vi "Autonomous Independent.vi"() -> ()   [LabVIEW 2014]
doc: "This VI is called when autonomous begins, and will automatically be terminated when autonomous ends. You can carry out timed or sensor driven robot movement independently without needing to return to the caller."
uses:
  Command Type.ctl
  <vilib>/Rock Robotics/WPI/RobotDrive/WPI_RobotDriveDevRef.ctl
  <vilib>/Rock Robotics/WPI/MotorControl/WPI_MotorControlDeviceRef.ctl
  <vilib>/Rock Robotics/WPI/MotorControl/WPI_MotorControlType.ctl
  <vilib>/Rock Robotics/SystemInterfaces/Typedef/FPGA_TypedefDigitalModule.ctl
  <vilib>/Rock Robotics/SystemInterfaces/DIO/FPGA_DIOPWMChannel.ctl
  <vilib>/Rock Robotics/WPI/PWM/WPI_PWMDeadband.ctl
  <vilib>/Rock Robotics/WPI/CAN/Jaguar/SubVIs/WPI_CANJaguar_ControlMode.ctl
  <vilib>/Rock Robotics/WPI/CAN/TalonSRX/WPI_CANTalonSRX_APIControlMode.ctl
  <vilib>/Rock Robotics/WPI/PWM/WPI_PWMTransform_ConPane.ctl
  <vilib>/Rock Robotics/WPI/Encoder/WPI_EncoderDevRef.ctl
  <vilib>/Rock Robotics/SystemInterfaces/Encoder/FPGA_EncoderIdx.ctl
  <vilib>/Rock Robotics/SystemInterfaces/Counter/FPGA_CounterCtrSystemIndex.ctl
  <vilib>/Rock Robotics/WPI/Encoder/WPI_EncoderType.ctl
  Nav6Library/Nav6DevRef.ctl
  <vilib>/Rock Robotics/WPI/SerialPort/WPI_SerialPortRef.ctl
  Nav6Library/Nav6Mode.ctl
  <vilib>/addons/control/pid/pid.llb/PID Structure.ctl
  <vilib>/Rock Robotics/WPI/RobotDrive/WPI_RobotDriveGetSetRefNum.vi
  <vilib>/Rock Robotics/Network Tables/SD Read Number.vi
  Robot Global Data.vi
  <vilib>/Rock Robotics/Network Tables/SD Write String.vi
  <vilib>/addons/control/pid/pid.llb/PID (DBL).vi
  GyroGlobal.vi
  <vilib>/addons/control/pid/NI_PID_pid.lvlib
  Nav6Library/Nav6.lvlib
  <vilib>/addons/control/pid/pid.llb/PID Structure Conversion (DBL).vi
  <vilib>/ptbypt/NI_PtbyPt.lvlib
panel:
  in  "stop 3":bool
  out "Outputs 2":dbl(graph)
  in  "Auton Routines":T1[](array[typedef])
  in  "Debug":bool
  in  "stop 2":bool
  in  "stop":bool
  out "Encoders":cluster{dbl, "Distance":dbl, "Distance":dbl}(graph)
  out "Outputs":T2(graph)
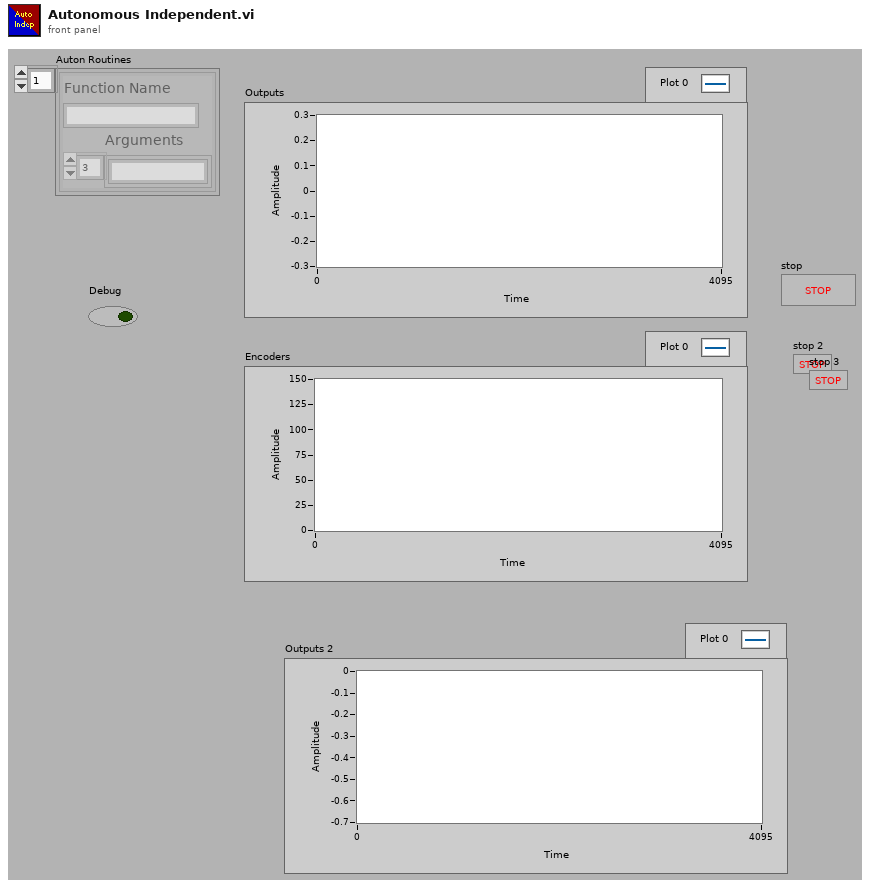
[diagram p1: front panel]
types:
  T1 = typedef "Command Type.ctl" = cluster{"Function Name":string, "Arguments":string[]}
  T2 = cluster{"Motor Values[0]":dbl, "Motor Values[1]":dbl}
  T3 = typedef "WPI_RobotDriveDevRef.ctl" = cluster{"DevStatus":errorcluster, "Motors[]":T4[], "Square Inputs":bool, "Max Output":dbl}
  T4 = typedef "WPI_MotorControlDeviceRef.ctl" = cluster{"DeviceStatus":errorcluster, "Type":T5, "PWM":cluster{"Controller":T6, "PWM Channel":T7, "DeadBand":T8}, "CAN":cluster{"Device Number":u8, "Control Mode":T9, "Semaphore":T10, "Max Vout":dbl, "TalonSRX Control Mode":T11}, "Invert":bool, "TransformRef":T12, "InvTransformRef":T12}
  T5 = typedef "WPI_MotorControlType.ctl" = enum16{"PWM", "CAN", "CANTalonSRX"}
  T6 = typedef "FPGA_TypedefDigitalModule.ctl" = enum16{"Controller 1"}
  T7 = typedef "FPGA_DIOPWMChannel.ctl" = enum8{"PWM 0", "PWM 1", "PWM 2", "PWM 3", "PWM 4", "PWM 5", "PWM 6", "PWM 7", "PWM 8", "PWM 9", "PWM MXP 0", "PWM MXP 1", "PWM MXP 2", "PWM MXP 3", "PWM MXP 4", "PWM MXP 5", "PWM MXP 6", "PWM MXP 7", "PWM MXP 8", "PWM MXP 9", "Invalid"}
  T8 = typedef "WPI_PWMDeadband.ctl" = cluster{"Name":string, "maxPositivePwm":i32, "minPositivePwm":i32, "centerPwm":i32, "maxNegativePwm":i32, "minNegativePwm":i32, "angularRange":u16}
  T9 = typedef "WPI_CANJaguar_ControlMode.ctl" = enum8{"Percent VBus", "Current", "Speed", "Position", "Voltage"}
  T10 = typedef "Semaphore RefNum" = refnum<k1>
  T11 = typedef "WPI_CANTalonSRX_APIControlMode.ctl" = enum8{"Percent VBus", "Speed", "Position", "Slave", "Unchanged / Invalid"}
  T12 = typedef "WPI_PWMTransform_ConPane.ctl" = refnum<vi>
  T13 = typedef "WPI_EncoderDevRef.ctl" = cluster{"DevStatus":errorcluster, "EncoderIndex":T14, "CounterIndex":T15, "DistancePerCount":dbl, "Decoding Type":T16}
  T14 = typedef "FPGA_EncoderIdx.ctl" = enum8{"Enc 0", "Enc 1", "Enc 2", "Enc 3", "Enc 4", "Enc 5", "Enc 6", "Enc 7", "Invalid"}
  T15 = typedef "FPGA_CounterCtrSystemIndex.ctl" = enum8{"Ctr 0", "Ctr 1", "Ctr 2", "Ctr 3", "Ctr 4", "Ctr 5", "Ctr 6", "Ctr 7", "Invalid"}
  T16 = typedef "WPI_EncoderType.ctl" = enum16{"1x", "2x", "4x"}
  T17 = typedef "Nav6.lvlib/Nav6DevRef.ctl" = cluster{"SerialPortRef":T18, "UpdateRate":u8, "Error":errorcluster, "Nav6Mode":T19}
  T18 = typedef "WPI_SerialPortRef.ctl" = cluster{"DevStatus":errorcluster, "Serial Port Name":refnum<visa-resource-name>}
  T19 = typedef "Nav6.lvlib/Nav6Mode.ctl" = enum16{"YPR", "Gyro", "Quaternion"}
  T20 = cluster{"Motors":T3, "EncoderR":T13, "EncoderL":T13, "Nav6":T17}
  T21 = typedef "NI_PID_pid.lvlib/PID Structure.ctl" = u16
  T22 = cluster{"proportional gain (Kc)":dbl, "integral time (Ti, min)":dbl, "derivative time (Td, min)":dbl}
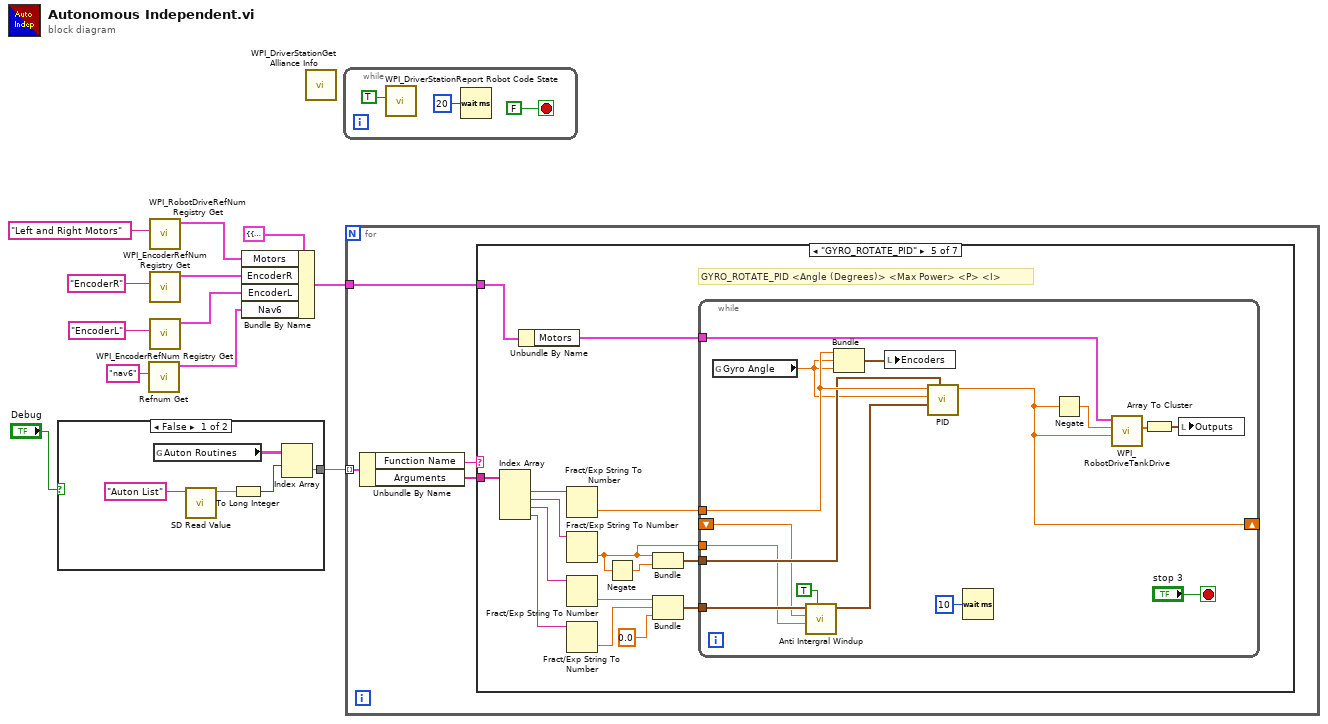
[diagram p0: block diagram]
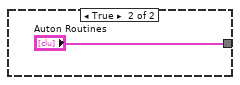
[diagram p2: hidden frame]
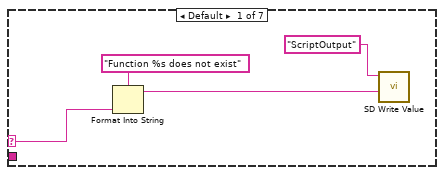
[diagram p3: hidden frame]
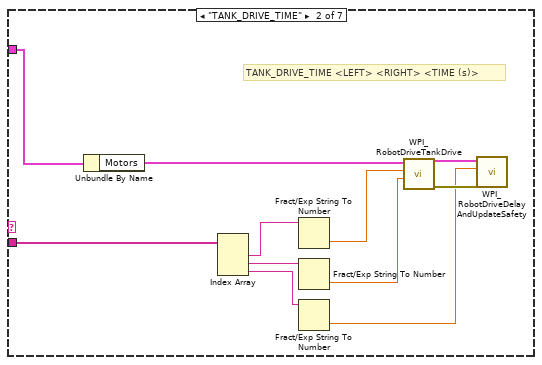
[diagram p4: hidden frame]
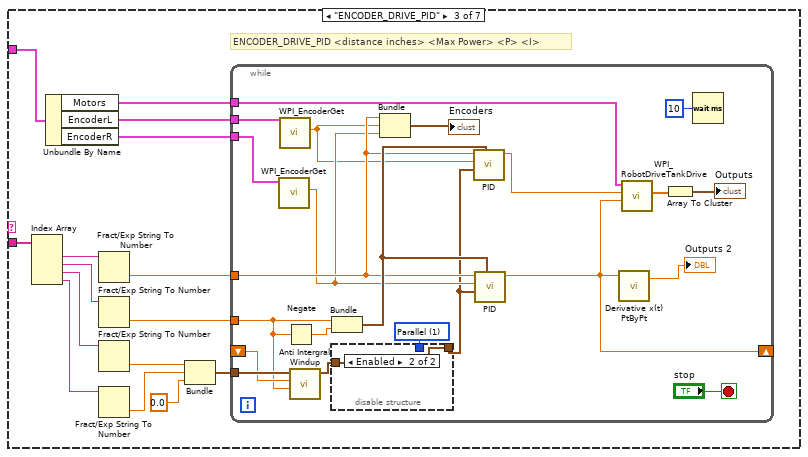
[diagram p5: hidden frame]
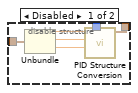
[diagram p6: hidden frame]
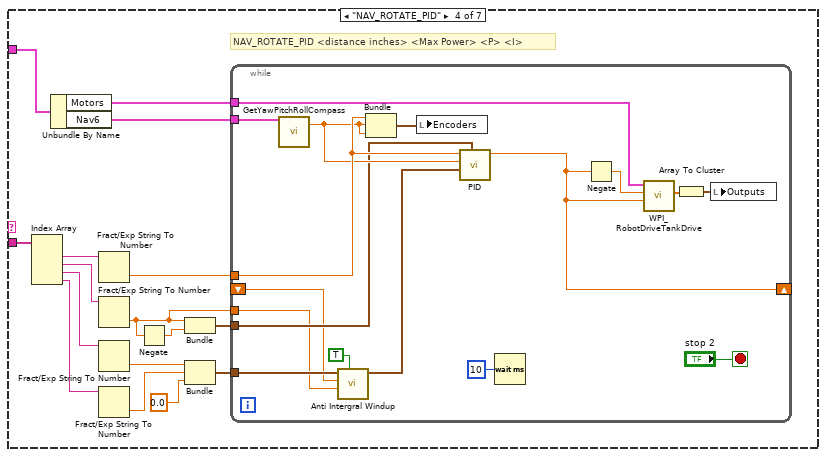
[diagram p7: hidden frame]
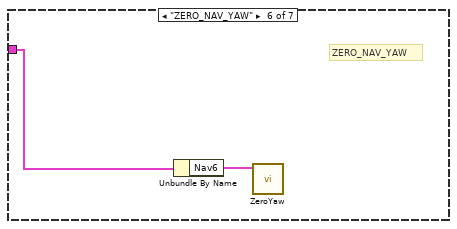
[diagram p8: hidden frame]
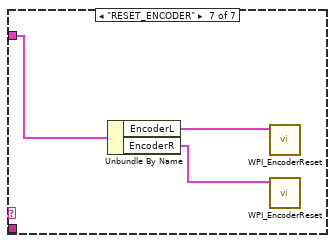
[diagram p9: hidden frame]
diagram:
  n1 = case shown="False" "Debug" {
    tunnel: [w13 "Auton Routines"] -> w12
    frame False {
      n2 = global read "Robot Global Data.vi" "Auton Routines"() -> (w16:T1[][])
      n3 = call-poly <vilib>:"SD Read Value.vi"("Name"="Auton List") -> ("Numeric"=w14:dbl)  [unwired: 8 in, 2 out]
      n4 = To Long Integer(number=w14) -> (32bit integer=w17:i32)
      n5 = Index Array(array=w16, index (row)=w17) -> (element=w13:T1[])  [unwired: 1 in]
    }
    frame True {
    }
  }
  n6 = call "Refnum Get.vi"("refnum name"="nav6") -> ("Nav6DevRef"=w2:T17)  [unwired: 9 in, 1 out]
  n7 = call <vilib>:"WPI_RobotDriveRefNum Registry Get.vi"("refnum name"="Left and Right Motors") -> ("RobotDriveDevRef"=w6:T3)  [unwired: 9 in, 1 out]
  n8 = call <vilib>:"WPI_EncoderRefNum Registry Get.vi"("refnum name"="EncoderR") -> ("EncoderDevRef"=w7:T13)  [unwired: 9 in, 1 out]
  n9 = call <vilib>:"WPI_EncoderRefNum Registry Get.vi"("refnum name"="EncoderL") -> ("EncoderDevRef"=w8:T13)  [unwired: 9 in, 1 out]
  n10 = Bundle By Name(cluster=T20 {"Motors"={"DevStatus"={"status"=FALSE, "code"=0, "source"=""}, "Motors[]"=[], "Square Inputs"=FALSE, "Max Output"=1.0}, "EncoderR"={"DevStatus"={"status"=FALSE, "code"=0, "source"=""}, "EncoderIndex"=enum."Invalid", "CounterIndex"=enum."Invalid", "DistancePerCount"=1.0, "Decoding Type"=enum."4x"}, "EncoderL"={"DevStatus"={"status"=FALSE, "code"=0, "source"=""}, "EncoderIndex"=enum."Invalid", "CounterIndex"=enum."Invalid", "DistancePerCount"=1.0, "Decoding Type"=enum."4x"}, "Nav6"={"SerialPortRef"={"DevStatus"={"status"=FALSE, "code"=0, "source"=""}, "Serial Port Name"=""}, "UpdateRate"=0, "Error"={"status"=FALSE, "code"=0, "source"=""}, "Nav6Mode"=enum."YPR"}}, "Motors"=w6, "EncoderR"=w7, "EncoderL"=w8, "Nav6"=w2) -> (w4:T20)
  n11 = call <vilib>:"WPI_DriverStationGet Alliance Info.vi"() -> ()  [unwired: 12 out]
  n12 = while {
    stop <- FALSE stop-if-true
    n13 = call <vilib>:"WPI_DriverStationReport Robot Code State.vi"("Autonomous"=TRUE) -> ()  [unwired: 10 in, 1 out]
    n14 = Wait (ms)(milliseconds to wait=u32 20) -> ()  [unwired: 1 out]
  }
  n15 = for {
    tunnel: w12 -> [w25] mode=indexing
    tunnel: w4 -> [w22]
    n16 = Unbundle By Name(w25) -> ("Function Name"=w24:string, "Arguments"=w23:string[])
    n17 = case shown="\"GYRO_ROTATE_PID\"" w24 {
      selector: w24 -> [w28 _ _ _ _ _ _]
      tunnel: w23 -> [_ w38 w55 w100 w132 _ _]
      tunnel: w22 -> [_ w31 w50 w96 w128 w150 w153]
      frame Default {
        n18 = Format Into String(format string="Function %s does not exist", w28) -> (resulting string=w26:string)  [unwired: 2 in, 1 out]
        n19 = call-poly <vilib>:"SD Write Value.vi"("String"=w26, "Name"="ScriptOutput") -> ()  [unwired: 8 in, 2 out]
      }
      frame "TANK_DRIVE_TIME" {
        # "TANK_DRIVE_TIME <LEFT> <RIGHT> <TIME (s)>"
        n20 = Unbundle By Name(w31) -> ("Motors"=w30:T3)
        n21 = Index Array(array=w38) -> (element #1=w37:string, element #2=w36:string, element #3=w35:string)  [unwired: 3 in]
        n22 = Fract/Exp String To Number(string=w37) -> (number=w34:dbl)  [unwired: 3 in, 1 out]
        n23 = Fract/Exp String To Number(string=w36) -> (number=w33:dbl)  [unwired: 3 in, 1 out]
        n24 = Fract/Exp String To Number(string=w35) -> (number=w32:dbl)  [unwired: 3 in, 1 out]
        n25 = call <vilib>:"WPI_RobotDriveTankDrive.vi"("Right axis value"=w33, "Left axis value"=w34, "RobotDriveDevRef"=w30) -> ("error out"=w40:errorcluster, "RobotDriveDevRef"=w39:T3)  [unwired: 6 in, 1 out]
        n26 = call <vilib>:"WPI_RobotDriveDelayAndUpdateSafety.vi"("error in (no error)"=w40, "Delay (s)"=w32, "RobotDriveDevRef"=w39) -> ()  [unwired: 7 in, 2 out]
      }
      frame "ENCODER_DRIVE_PID" {
        # "ENCODER_DRIVE_PID <distance inches> <Max Power> <P> <I>"
        n27 = Index Array(array=w55) -> (element #1=w53:string, element #2=w54:string, element #3=w46:string, element #4=w45:string)  [unwired: 4 in]
        n28 = Unbundle By Name(w50) -> ("Motors"=w47:T3, "EncoderL"=w48:T13, "EncoderR"=w49:T13)
        n29 = Fract/Exp String To Number(string=w53) -> (number=w52:dbl)  [unwired: 3 in, 1 out]
        n30 = Fract/Exp String To Number(string=w54) -> (number=w51:dbl)  [unwired: 3 in, 1 out]
        n31 = Fract/Exp String To Number(string=w46) -> (number=w44:dbl)  [unwired: 3 in, 1 out]
        n32 = Fract/Exp String To Number(string=w45) -> (number=w43:dbl)  [unwired: 3 in, 1 out]
        n33 = Bundle(w44, w43, 0.0) -> (w42:cluster{dbl, dbl, dbl})  [unwired: 1 in]
        n34 = while {
          tunnel: w52 -> [w69]
          tunnel: w51 -> [w60]
          tunnel: w49 -> [w75]
          tunnel: w48 -> [w74]
          tunnel: w47 -> [w73]
          tunnel: w42 -> [w62]
          shift-right: [w63] -> _
          shift-left: _ -> [w61]
          stop <- "stop" stop-if-true
          w57 = T21 1 items=["Academic (Standard)", "Parallel", "Series"] ("PID structure")
          n35 = call <vilib>:"WPI_EncoderGet.vi"("EncoderDevRef"=w75) -> ("Distance"=w68:dbl)  [unwired: 5 in, 5 out]
          n36 = call <vilib>:"WPI_EncoderGet.vi"("EncoderDevRef"=w74) -> ("Distance"=w65:dbl)  [unwired: 5 in, 5 out]
          n37 = Negate(x=w60) -> (-x=w77:dbl)
          n38 = call "Anti Intergral Windup.vi"("|Limit|"=w60, "MV"=w61, "PID gains"=w62) -> ("PID gains"=w58:T22)  [unwired: 8 in]
          n39 = Bundle(w60, w77) -> (w76:cluster{dbl, dbl})  [unwired: 1 in]
          n40 = disable-structure shown="Enabled" {
            disable-tunnel: [w83 w84] -> w59
            disable-tunnel: w58 -> [w82 w84]
            disable-tunnel: w57 -> [w78 _]
            frame Disabled {
              n41 = Unbundle(w82) -> ("proportional gain (Kc)"=w81:dbl, "integral time (Ti, min)"=w80:dbl, "derivative time (Td, min)"=w79:dbl)
              n42 = call-poly <vilib>:"PID Structure Conversion.vi"("PID structure"=w78, "derivative"=w79, "integral"=w80, "proportional"=w81) -> ("PID gains"=w83:T22)  [unwired: 7 in]
            }
            frame Enabled {
            }
          }
          n43 = Bundle(w69, "Distance"=w65, "Distance"=w68) -> (→"Encoders":cluster{dbl, "Distance":dbl, "Distance":dbl})  [unwired: 1 in]
          n44 = call-poly <vilib>:"PID.vi"("output range"=w76, "PID gains"=w59, "process variable"=w65, "setpoint"=w69) -> ("output"=w64:dbl)  [unwired: 6 in, 1 out]
          n45 = call-poly <vilib>:"PID.vi"("output range"=w76, "PID gains"=w59, "process variable"=w68, "setpoint"=w69) -> ("output"=w63:dbl)  [unwired: 6 in, 1 out]
          n46 = call <vilib>:"Derivative x(t) PtByPt.vi"("x"=w63) -> ("dx/dt"=→"Outputs 2":dbl)  [unwired: 3 in, 1 out]
          n47 = call <vilib>:"WPI_RobotDriveTankDrive.vi"("Right axis value"=w63, "Left axis value"=w64, "RobotDriveDevRef"=w73) -> ("Motor Values"=w72:dbl[])  [unwired: 6 in, 2 out]
          n48 = Array To Cluster(array=w72) -> (cluster=→"Outputs":T2)
          n49 = Wait (ms)(milliseconds to wait=u32 10) -> ()  [unwired: 1 out]
        }
      }
      frame "NAV_ROTATE_PID" {
        # "NAV_ROTATE_PID <distance inches> <Max Power> <P> <I>"
        n50 = Index Array(array=w100) -> (element #1=w98:string, element #2=w99:string, element #3=w94:string, element #4=w93:string)  [unwired: 4 in]
        n51 = Unbundle By Name(w96) -> ("Motors"=w95:T3, "Nav6"=w88:T17)
        n52 = Fract/Exp String To Number(string=w98) -> (number=w97:dbl)  [unwired: 3 in, 1 out]
        n53 = Fract/Exp String To Number(string=w99) -> (number=w85:dbl)  [unwired: 3 in, 1 out]
        n54 = Fract/Exp String To Number(string=w94) -> (number=w92:dbl)  [unwired: 3 in, 1 out]
        n55 = Fract/Exp String To Number(string=w93) -> (number=w91:dbl)  [unwired: 3 in, 1 out]
        n56 = Negate(x=w85) -> (-x=w87:dbl)
        n57 = Bundle(w85, w87) -> (w86:cluster{dbl, dbl})  [unwired: 1 in]
        n58 = Bundle(w92, w91, 0.0) -> (w90:cluster{dbl, dbl, dbl})  [unwired: 1 in]
        n59 = while {
          tunnel: w97 -> [w115]
          tunnel: w95 -> [w117]
          tunnel: w90 -> [w105]
          tunnel: w88 -> [w111]
          tunnel: w86 -> [w106]
          shift-right: [w113] -> _
          shift-left: _ -> [w103]
          tunnel: w85 -> [w102]
          stop <- "stop 2" stop-if-true
          n60 = call "GetYawPitchRollCompass.vi"("Nav6DevRef"=w111) -> ("Yaw"=w107:dbl)  [unwired: 12 in, 6 out]
          n61 = call "Anti Intergral Windup.vi"("Disable"=TRUE, "|Limit|"=w102, "MV"=w103, "PID gains"=w105) -> ("PID gains"=w104:T22)  [unwired: 7 in]
          n62 = Bundle(w115, "Yaw"=w107, "Yaw"=w107) -> (w110:cluster{dbl, "Yaw":dbl, "Yaw":dbl})  [unwired: 1 in]
          n63 = local write "Encoders"(w110) -> ()
          n64 = call-poly <vilib>:"PID.vi"("output range"=w106, "PID gains"=w104, "process variable"=w107, "setpoint"=w115) -> ("output"=w113:dbl)  [unwired: 6 in, 1 out]
          n65 = Wait (ms)(milliseconds to wait=u32 10) -> ()  [unwired: 1 out]
          n66 = Negate(x=w113) -> (-x=w108:dbl)
          n67 = call <vilib>:"WPI_RobotDriveTankDrive.vi"("Right axis value"=w113, "Left axis value"=w108, "RobotDriveDevRef"=w117) -> ("Motor Values"=w116:dbl[])  [unwired: 6 in, 2 out]
          n68 = Array To Cluster(array=w116) -> (cluster=w112:T2)
          n69 = local write "Outputs"(w112) -> ()
        }
      }
      frame "GYRO_ROTATE_PID" {
        # "GYRO_ROTATE_PID <Angle (Degrees)> <Max Power> <P> <I>"
        n70 = Index Array(array=w132) -> (element #1=w130:string, element #2=w131:string, element #3=w126:string, element #4=w125:string)  [unwired: 4 in]
        n71 = Unbundle By Name(w128) -> ("Motors"=w127:T3)
        n72 = Fract/Exp String To Number(string=w130) -> (number=w129:dbl)  [unwired: 3 in, 1 out]
        n73 = Fract/Exp String To Number(string=w131) -> (number=w118:dbl)  [unwired: 3 in, 1 out]
        n74 = Fract/Exp String To Number(string=w126) -> (number=w124:dbl)  [unwired: 3 in, 1 out]
        n75 = Fract/Exp String To Number(string=w125) -> (number=w123:dbl)  [unwired: 3 in, 1 out]
        n76 = Negate(x=w118) -> (-x=w120:dbl)
        n77 = Bundle(w118, w120) -> (w119:cluster{dbl, dbl})  [unwired: 1 in]
        n78 = Bundle(w124, w123, 0.0) -> (w122:cluster{dbl, dbl, dbl})  [unwired: 1 in]
        n79 = while {
          tunnel: w129 -> [w146]
          tunnel: w127 -> [w148]
          tunnel: w122 -> [w139]
          tunnel: w119 -> [w140]
          shift-right: [w144] -> _
          shift-left: _ -> [w137]
          tunnel: w118 -> [w136]
          stop <- "stop 3" stop-if-true
          n80 = global read "GyroGlobal.vi" "Gyro Angle"() -> (w134:dbl)
          n81 = call "Anti Intergral Windup.vi"("Disable"=TRUE, "|Limit|"=w136, "MV"=w137, "PID gains"=w139) -> ("PID gains"=w138:T22)  [unwired: 7 in]
          n82 = Bundle(w146, "Gyro Angle"=w134, "Gyro Angle"=w134) -> (w133:cluster{dbl, "Gyro Angle":dbl, "Gyro Angle":dbl})  [unwired: 1 in]
          n83 = local write "Encoders"(w133) -> ()
          n84 = call-poly <vilib>:"PID.vi"("output range"=w140, "PID gains"=w138, "process variable"=w134, "setpoint"=w146) -> ("output"=w144:dbl)  [unwired: 6 in, 1 out]
          n85 = Wait (ms)(milliseconds to wait=u32 10) -> ()  [unwired: 1 out]
          n86 = Negate(x=w144) -> (-x=w141:dbl)
          n87 = call <vilib>:"WPI_RobotDriveTankDrive.vi"("Right axis value"=w144, "Left axis value"=w141, "RobotDriveDevRef"=w148) -> ("Motor Values"=w147:dbl[])  [unwired: 6 in, 2 out]
          n88 = Array To Cluster(array=w147) -> (cluster=w143:T2)
          n89 = local write "Outputs"(w143) -> ()
        }
      }
      frame "ZERO_NAV_YAW" {
        # "ZERO_NAV_YAW"
        n90 = Unbundle By Name(w150) -> ("Nav6"=w149:T17)
        n91 = call "ZeroYaw.vi"("Nav6DevRef"=w149) -> ()  [unwired: 9 in, 2 out]
      }
      frame "RESET_ENCODER" {
        n92 = Unbundle By Name(w153) -> ("EncoderL"=w152:T13, "EncoderR"=w151:T13)
        n93 = call <vilib>:"WPI_EncoderReset.vi"("EncoderDevRef"=w152) -> ()  [unwired: 9 in, 2 out]
        n94 = call <vilib>:"WPI_EncoderReset.vi"("EncoderDevRef"=w151) -> ()  [unwired: 9 in, 2 out]
      }
    }
  }
